vi "PackageNode_Create.vi"(0 "reference":refnum<class "PackageNode.lvclass">, 5 "error in (no error)":errorcluster, 6 "GoopReferenceIn":T1) -> (14 "reference out":refnum<class "PackageNode.lvclass">, 16 "# of objects":i32, 19 "error out":errorcluster)   [LabVIEW 2014, in "PackageNode.lvclass"]
doc: "Creates and initializes a new PackageNode object.\n\nThis object should be destroyed using a PackageNode destructor VI or a virtual base class destructor VI.\n\n[GOOP 2.1]"
uses:
  <resource>/Framework/Providers/Open_GDS/UML/PackageNode_class/PackageNode.lvclass
  <resource>/Framework/Providers/Open_GDS/UML/AbstractNode_class/ObjectReference.ctl
  <resource>/Framework/Providers/Open_GDS/UML/RectangularNode_class/RectangularNode.lvclass
  <resource>/Framework/Providers/Open_GDS/UML/MultiLineString_class/MultiLineString.lvclass
  <resource>/Framework/Providers/Open_GDS/UML/AbstractNode_class/AbstractNode.lvclass
panel:
  # "The input reference should only\nbe wired when this method is called\nby a sub class constructor."
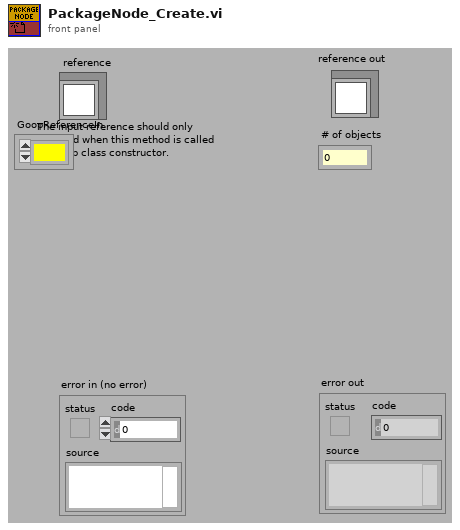
[diagram p1: front panel]
types:
  T1 = typedef "AbstractNode.lvclass/ObjectReference.ctl" = refnum<k1>
  T2 = typedef "PackageNode.lvclass/ObjectAttributes.ctl" = cluster{"Base class":T3, "name":string, "contents":refnum<class "MultiLineString.lvclass">, "DEFAULT_TOP_WIDTH":i32, "DEFAULT_TOP_HEIGHT":i32, "DEFAULT_WIDTH":i32, "DEFAULT_HEIGHT":i32, "NAME_GAP":i32, "XGAP":i32, "YGAP":i32, "Collapsed":bool, "Note color":u32, "Justification":u16}
  T3 = typedef "RectangularNode.lvclass/ObjectAttributes.ctl" = cluster{"Base class":T4, "bounds":T5}
  T4 = typedef "AbstractNode.lvclass/ObjectAttributes.ctl" = cluster{"parent":refnum<class "AbstractNode.lvclass">, "children":refnum<class "AbstractNode.lvclass">[], "Hidden":bool}
  T5 = typedef "Rectangle Rectangle2D.ctl" = cluster{"x":dbl, "y":dbl, "width":dbl, "height":dbl}
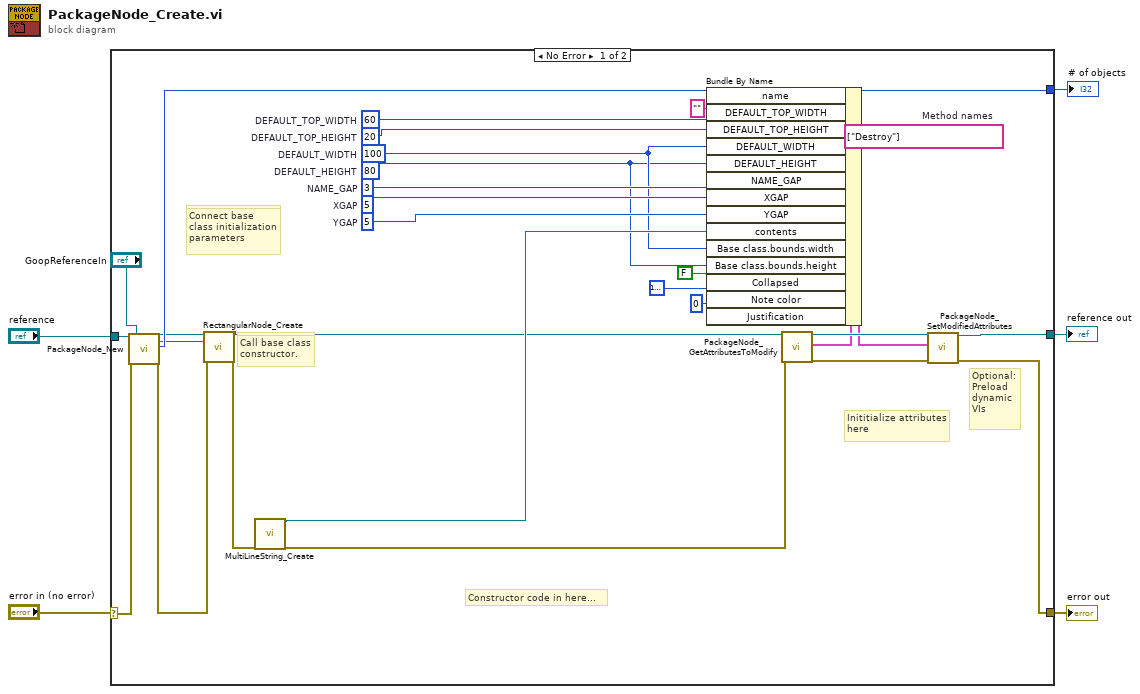
[diagram p0: block diagram]
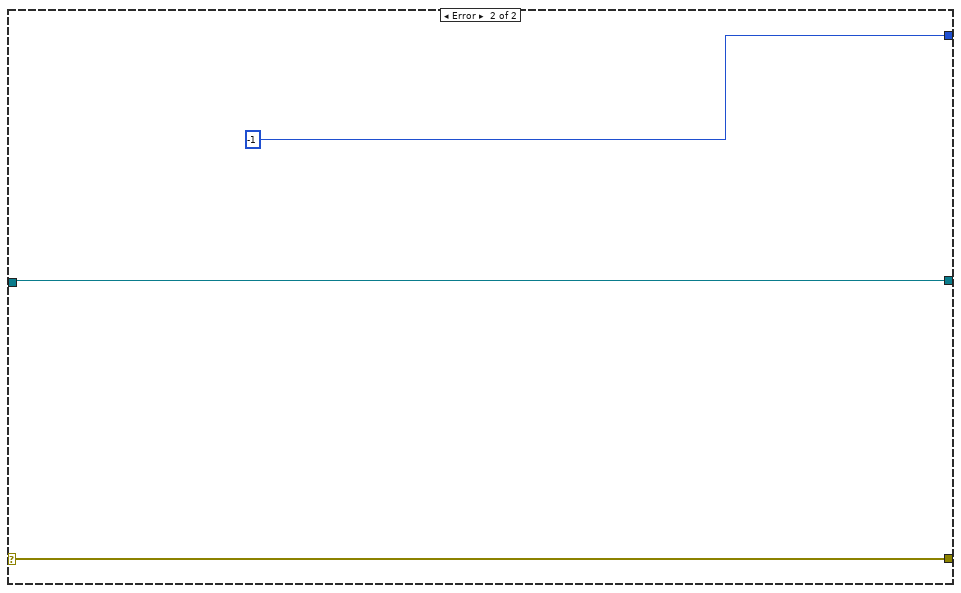
[diagram p2: hidden frame]
diagram:
  n1 = case shown="No Error" "error in (no error)" {
    selector: "error in (no error)" -> [w33 w35]
    tunnel: [w26 w34] -> w5
    tunnel: [w25 w35] -> w4
    tunnel: [w32 -1 ("Nr of open handles")] -> w3
    tunnel: "reference" -> [w31 w34]
    frame No Error {
      (unwired) string[] ["Destroy"]  # Method names
      w17 = 5  # YGAP
      w18 = 5  # XGAP
      w19 = 3  # NAME_GAP
      w12 = 80  # DEFAULT_HEIGHT
      w13 = 100  # DEFAULT_WIDTH
      w20 = 20  # DEFAULT_TOP_HEIGHT
      w21 = 60  # DEFAULT_TOP_WIDTH
      # "Connect base\nclass initialization\nparameters"
      # "Call base class\nconstructor."
      # "Optional:\nPreload\ndynamic\nVIs"
      # "Connect base\nclass initialization\nparameters"
      # "Inititialize attributes\nhere"
      # "Constructor code in here..."
      # "Call base class\nconstructor."
      n2 = call <resource>:"PackageNode_New.vi"("reference in"=w31, "error in (no error)"=w33, "GoopReferenceIn"="GoopReferenceIn") -> ("GoopReferenceOut"=w9:T1, "reference out"=w28:refnum<class "PackageNode.lvclass">, "# of objects"=w32:i32, "error out"=w30:errorcluster)  [unwired: 2 in, 11 out]
      n3 = call <resource>:"RectangularNode_Create.vi"("reference"=w28, "error in (no error)"=w30, "GoopReferenceIn"=w9) -> ("reference out"=w11:refnum<class "PackageNode.lvclass">, "error out"=w24:errorcluster)  [unwired: 15 out]
      n4 = call <resource>:"MultiLineString_Create.vi"("error in (no error)"=w24) -> ("reference out"=w15:refnum<class "MultiLineString.lvclass">, "error out"=w16:errorcluster)  [unwired: 3 in, 14 out]
      n5 = call <resource>:"PackageNode_GetAttributesToModify.vi"("reference in"=w11, "error in (no error)"=w16) -> ("reference out"=w27:refnum<class "PackageNode.lvclass">, "Attributes"=w22:T2, "error out"=w29:errorcluster)  [unwired: 1 in, 14 out]
      n6 = Bundle By Name(cluster=w22, "name"="", "DEFAULT_TOP_WIDTH"=w21, "DEFAULT_TOP_HEIGHT"=w20, "DEFAULT_WIDTH"=w13, "DEFAULT_HEIGHT"=w12, "NAME_GAP"=w19, "XGAP"=w18, "YGAP"=w17, "contents"=w15, "Base class.bounds.width"=w13, "Base class.bounds.height"=w12, "Collapsed"=FALSE, "Note color"=u32 16777216, "Justification"=u16 0) -> (w23:T2)
      n7 = call <resource>:"PackageNode_SetModifiedAttributes.vi"("reference in"=w27, "Attributes"=w23, "error in (no error)"=w29) -> ("reference out"=w26:refnum<class "PackageNode.lvclass">, "error out"=w25:errorcluster)  [unwired: 3 in, 12 out]
    }
    frame Error {
    }
  }
  "error out" <- w4
  "reference out" <- w5
  "# of objects" <- w3
